vi "Configure_Gill.vi"(0 "Analogue O/P Config":u16(ring) items=["0 to 5 volt", "+/-2.5 Volt", "4-20mA"], 1 "ORIGINAL Address":u8=66 min=65 max=90, 2 "NEW Address":u8=66 min=65 max=90, 5 "Analogue O/P Scale":u16(ring) items=["10m/s", "20m/s", "30m/s", "40m/s", "50m/s", "60m/s", "70m/s"], 7 "Averaging Time":u16(ring)=3 items=["OFF", "3 seconds", "5 seconds", "10 seconds"], 9 "Samples/sec":u16(ring) items=["1 sample/sec", "4 samples/sec"], 12 "Port Name":string="Edge0164-P2") -> ()   [LabVIEW 2011]
panel:
  out "Read":string="\r\n\r\nCONFIGURATION MODE\r\nM4\r\nM4\r\nU1\r\nU1\r\nG4\r\nG4\r\nO2\r\nO2\r\nV1\r\nV1\r\nP1\r\nP1\r\nT1\r\nT1\r\nS1\r\nS1\r\nC1\r\nC1\r\nA1\r\nA1\r\nI2\r\nI2\r\nNB\r\nNB\r\nD3\r\ncurrent configuration :\r\nP1 G4 M4 U1 B3 F1 T1 S1 C1 I2 V1 A1 NB O2\r\nD3\r\nQ\r\nQ\r\n"
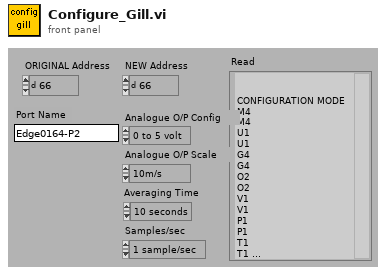
[diagram p1: front panel]
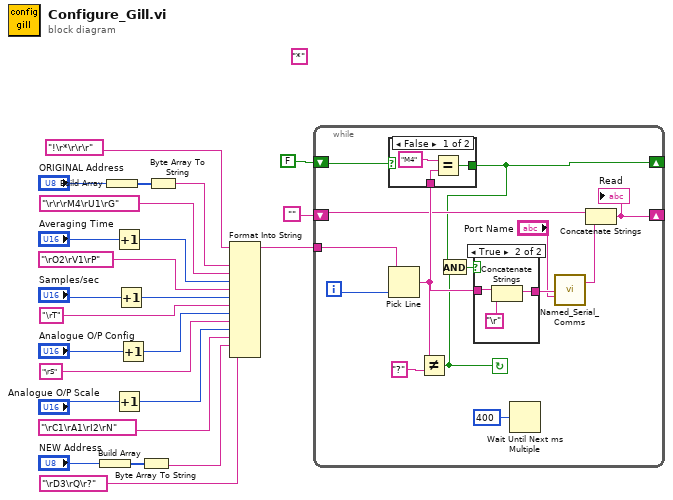
[diagram p0: block diagram]
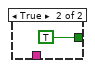
[diagram p2: hidden frame]
diagram:
  (unwired) "*"
  n1 = Build Array("NEW Address") -> (w14:u8[])
  n2 = Build Array("ORIGINAL Address") -> (w24:u8[])
  n3 = Increment(x="Averaging Time") -> (x+1=w18:u16)
  n4 = Increment(x="Analogue O/P Scale") -> (x+1=w4:u16)
  n5 = Increment(x="Samples/sec") -> (x+1=w16:u16)
  n6 = Increment(x="Analogue O/P Config") -> (x+1=w7:u16)
  n7 = Byte Array To String(unsigned byte array=w14) -> (string=w2:string)
  n8 = Byte Array To String(unsigned byte array=w24) -> (string=w20:string)
  n9 = Format Into String(initial string="!\r*\r\r\r", w20, "\r\r\rM4\rU1\rG", w18, "\rO2\rV1\rP", w16, "\rT", w7, "\rS", w4, "\rC1\rA1\rI2\rN", w2, "\rD3\rQ\r?") -> (resulting string=w21:string)  [unwired: 2 in, 1 out]
  n10 = while {
    shift-left: "" -> [w31]
    shift-right: [w30] -> _
    shift-left: FALSE -> [w33]
    shift-right: [w29] -> _
    tunnel: w21 -> [w38]
    i -> [w37]
    stop <- w27 continue-if-true
    n11 = Pick Line(multi-line string=w38, line index=w37) -> (output string=w35:string)  [unwired: 1 out]
    n12 = case shown="False" w33 {
      tunnel: w35 -> [w40 _]
      tunnel: [w39 TRUE] -> w29
      frame False {
        n13 = Equal?(x="M4", y=w40) -> (x = y?=w39:bool)
      }
      frame True {
      }
    }
    n14 = Not Equal?(x=w35, y="?") -> (x != y?=w27:bool)
    n15 = And(x=w29, y=w27) -> (x .and. y?=w28:bool)
    n16 = case shown="True" w28 {
      tunnel: [w43 w46] -> w34
      tunnel: w35 -> [w43 w45]
      frame False {
      }
      frame True {
        n17 = Concatenate Strings(w45, "\r") -> (w46:string)
      }
    }
    n18 = Wait Until Next ms Multiple(millisecond multiple=u32 400) -> ()  [unwired: 1 out]
    n19 = call "Named_Serial_Comms.vi"("Write String"=w34, "Port Name"="Port Name") -> ("Read"=w32:string)  [unwired: 7 in, 6 out]
    n20 = Concatenate Strings(w31, w32) -> (w30:string)
    "Read" <- w30
  }
